vi "TCPServer.vi"(8 "错误输入（无错误）":errorcluster, 10 "stop":bool) -> (0 "错误输出":errorcluster, 2 "members":i32 caption="members\non line")   [LabVIEW 2014]
panel:
  out "连接次数":i32
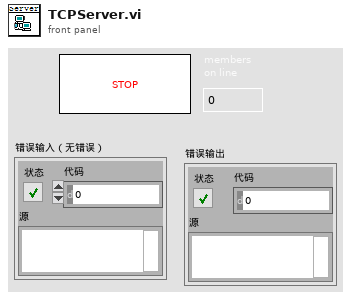
[diagram p1: front panel]
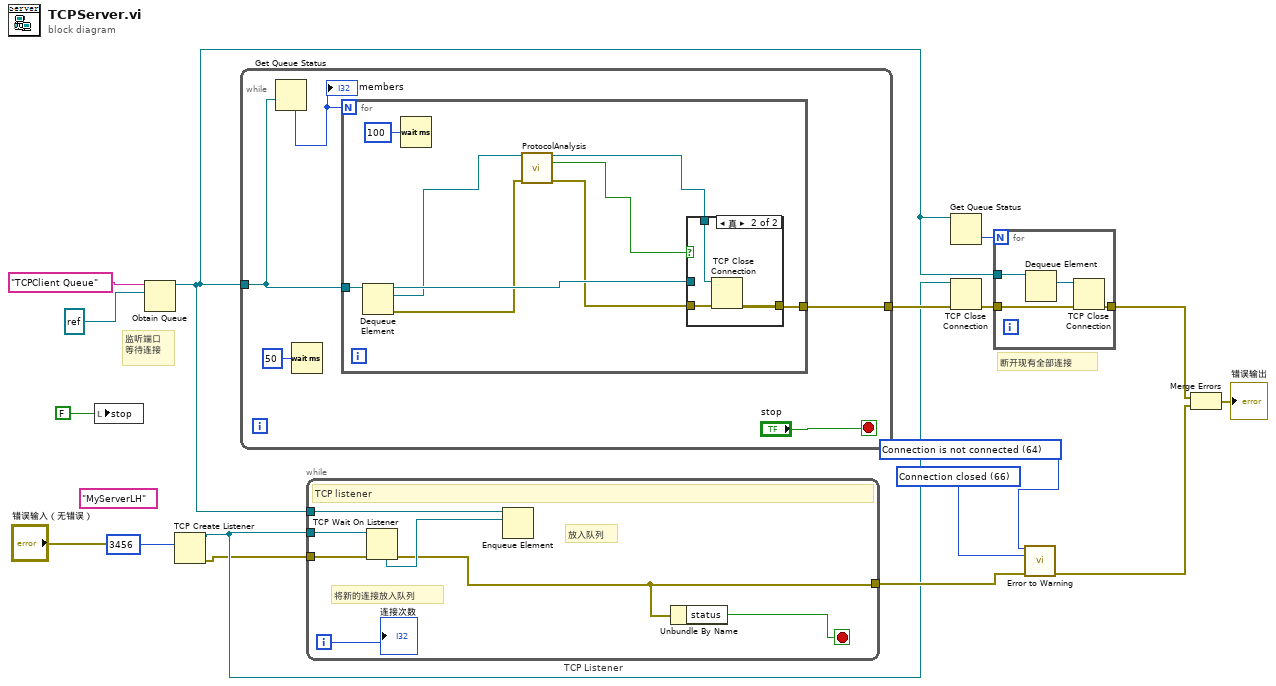
[diagram p0: block diagram]
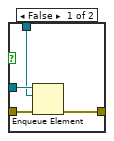
[diagram p2: hidden frame]
diagram:
  w1 = 66 items=["No Error", "Argument Error", "Memory Full", "Out of Zone", "End of File", "File Already Open", "Generic File IO Error", "File Not Found", "File Permission Error", "Disk Full", "Duplicate Path", "Too Many Files Open", "Not Enabled", "Resource File Not Found", "Cannot Add Resource", "Resource Not Found", "Image Not Found", "Image Memory Error", "Pen Does Not Exist", "Config Bad Type", "Config Token Not Found", "Config Parse Error", "Config Memory Error", "Bad External Code Format", "Bad External Code Offset", "External Code Not Present", "Null Window", "Destroy Window Mixup", "Null Menu", "Print Aborted", "Bad Print Record", "Print Driver Error", "Windows Error During Print", "Memory Error During Print", "Print Dialog Error", "Generic Print Error", "Invalid Device Refnum", "Device Not Found", "Device Parameter Error", "Device Unit Error", "Can't Open Device", "Device Call Aborted", "Generic Error", "Cancelled By User", "Object ID Too Low", "Object ID Too High", "Object Not In Heap", "Unknown Heap", "Bad DefProc ID", "DefProc Not In Table", "Message Out Of Range", "Null Method", "Unknown Message", "Manager Call Not Supported", "Bad address", "Connection In progress", "Connection timed out", "Connection is already in progress", "Network attribute not supported", "Network error", "Address in use", "System out of memory", "Connection aborted", "Connection refused", "Connection is not connected", "Connection is already connected", "Connection closed", "Initialize error (interapplication manager)", "Bad occurrence", "Wait on unbound occurrence handler", "Occurrence queue overflow", "Bad path", "Semaphore not signaled", "Unrecognized type (interapplication manager)"] ("2nd Error to Convert")
  w2 = 64 items=["No Error", "Argument Error", "Memory Full", "Out of Zone", "End of File", "File Already Open", "Generic File IO Error", "File Not Found", "File Permission Error", "Disk Full", "Duplicate Path", "Too Many Files Open", "Not Enabled", "Resource File Not Found", "Cannot Add Resource", "Resource Not Found", "Image Not Found", "Image Memory Error", "Pen Does Not Exist", "Config Bad Type", "Config Token Not Found", "Config Parse Error", "Config Memory Error", "Bad External Code Format", "Bad External Code Offset", "External Code Not Present", "Null Window", "Destroy Window Mixup", "Null Menu", "Print Aborted", "Bad Print Record", "Print Driver Error", "Windows Error During Print", "Memory Error During Print", "Print Dialog Error", "Generic Print Error", "Invalid Device Refnum", "Device Not Found", "Device Parameter Error", "Device Unit Error", "Can't Open Device", "Device Call Aborted", "Generic Error", "Cancelled By User", "Object ID Too Low", "Object ID Too High", "Object Not In Heap", "Unknown Heap", "Bad DefProc ID", "DefProc Not In Table", "Message Out Of Range", "Null Method", "Unknown Message", "Manager Call Not Supported", "Bad address", "Connection In progress", "Connection timed out", "Connection is already in progress", "Network attribute not supported", "Network error", "Address in use", "System out of memory", "Connection aborted", "Connection refused", "Connection is not connected", "Connection is already connected", "Connection closed", "Initialize error (interapplication manager)", "Bad occurrence", "Wait on unbound occurrence handler", "Occurrence queue overflow", "Bad path", "Semaphore not signaled", "Unrecognized type (interapplication manager)"] ("1st Error to Convert")
  (unwired) "MyServerLH" ("service name")
  # "监听端口\n等待连接"
  # "断开现有全部连接"
  n1 = local write "stop"(FALSE) -> ()
  n2 = Obtain Queue(name (unnamed)="TCPClient Queue" ("名称（未命名）"), element data type=refnum<k5> refnum ("connection ID")) -> (queue out=w13:refnum<queue>)  [unwired: 3 in, 2 out]
  n3 = TCP Create Listener(8:"错误输入（无错误）", 10:u16 3456 ("port")) -> (0:w6:errorcluster, 3:w7:refnum<k5>)  [unwired: 3 in, 1 out]
  n4 = while {
    tunnel: w13 -> [w22]
    tunnel: [w20] -> w12
    stop <- "stop" stop-if-true
    n5 = Get Queue Status(queue=w22) -> (# elements in queue=w19:i32)  [unwired: 2 in, 7 out]
    "members" <- w19
    n6 = Wait (ms)(milliseconds to wait=u32 50 ("等待时间（毫秒）")) -> ()  [unwired: 1 out]
    n7 = for {
      N: w19 -> [_]
      tunnel: w22 -> [w31]
      tunnel: [w29] -> w20
      n8 = Dequeue Element(queue=w31) -> (queue out=w30:refnum<queue>, element=w27:refnum<k5>, error out=w26:errorcluster)  [unwired: 2 in, 1 out]
      n9 = Wait (ms)(milliseconds to wait=u32 100 ("等待时间（毫秒）")) -> ()  [unwired: 1 out]
      n10 = call "ProtocolAnalysis.vi"("TCP ref in"=w27, "error in"=w26) -> ("TCP ref out"=w24:refnum<k5>, "Exit"=w23:bool, "error out"=w25:errorcluster)  [unwired: 11 in]
      n11 = case shown="真" w23 {
        tunnel: w30 -> [w35 _]
        tunnel: [w34 w38] -> w29
        tunnel: w25 -> [w33 w36]
        tunnel: w24 -> [w32 w37]
        frame False {
          n12 = Enqueue Element(queue=w35, element=w32, error in (no error)=w33) -> (error out=w34:errorcluster)  [unwired: 1 in, 2 out]
        }
        frame True {
          n13 = TCP Close Connection(connection ID=w37, error in (no error)=w36) -> (error out=w38:errorcluster)  [unwired: 1 in, 1 out]
        }
      }
    }
  }
  n14 = while "TCP Listener" {
    tunnel: w7 -> [w45]
    tunnel: w13 -> [w43]
    tunnel: w6 -> [w42]
    tunnel: [w41] -> w8
    i -> [w40]
    stop <- w39 stop-if-true
    # "放入队列"
    # "将新的连接放入队列"
    # "TCP listener"
    n15 = TCP Wait On Listener(8:w42, 11:w45) -> (0:w41:errorcluster, 4:w44:refnum<k5>)  [unwired: 2 in, 3 out]
    n16 = Enqueue Element(queue=w43, element=w44) -> ()  [unwired: 2 in, 3 out]
    n17 = Unbundle By Name(w41) -> ("status"=w39:bool)
    "连接次数" <- w40
  }
  n18 = Get Queue Status(queue=w13) -> (# elements in queue=w14:i32)  [unwired: 2 in, 7 out]
  n19 = TCP Close Connection(connection ID=w7, error in (no error)=w12) -> (error out=w15:errorcluster)  [unwired: 1 in, 1 out]
  n20 = for {
    N: w14 -> [_]
    tunnel: w15 -> [w49]
    tunnel: [w48] -> w10
    tunnel: w13 -> [w47]
    n21 = Dequeue Element(queue=w47) -> (element=w46:refnum<k5>)  [unwired: 2 in, 3 out]
    n22 = TCP Close Connection(connection ID=w46, error in (no error)=w49) -> (error out=w48:errorcluster)  [unwired: 1 in, 1 out]
  }
  n23 = call <vilib>:"Error to Warning.vi"("1st Error to Convert"=w2, "2nd Error to Convert"=w1, "error in"=w8) -> ("warning out"=w9:errorcluster)  [unwired: 12 in]
  n24 = Merge Errors(w10, w9) -> (→"错误输出":errorcluster)
